vi "Actor Core.vi"(8 "error in":errorcluster, 11 "Nested in":refnum<class "UI.lvclass">) -> (0 "error out":errorcluster, 3 "Actor out":refnum<class "Actor.lvclass">)   [LabVIEW 2020, in "UI.lvlib" / "UI.lvclass"]
doc: "(<B>Filename</B>: Actor Framework.lvlib:Actor.lvclass:Actor Core.vi)\n\nReceives messages to the actor, reacts to them, and initiates any error handling that may shut the actor down.\n\nDescendant classes may override this VI to append parallel tasks for the actor to complete while it handles messages. Overrides use the Call Parent Method node."
uses:
  UI.lvclass
  <vilib>/ActorFramework/Actor/Actor.lvclass
  <vilib>/ActorFramework/Stop Msg/Stop Msg.lvclass
  Monedas/Monedas.lvclass
  Productos/Productos.lvclass
  Mensajes/Mensajes.lvclass
panel:
  out "String":string
  out "Dinero 2":dbl
  out "Dinero":dbl
  out "Costo":dbl
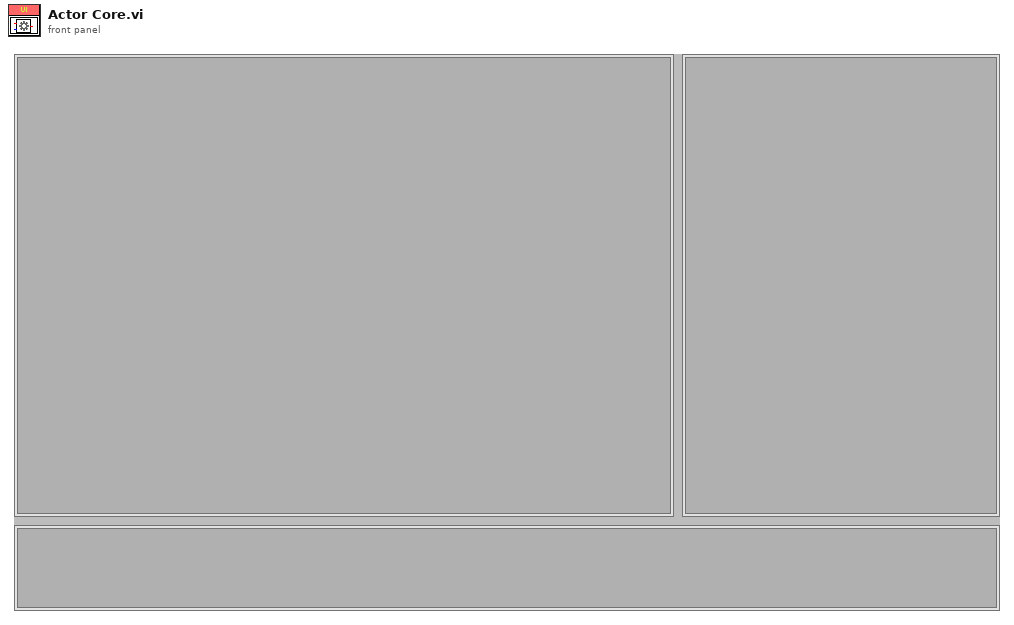
[diagram p1: front panel]
types:
  T1 = cluster{"Stop":refnum<user-event>, "Costo":refnum<user-event>, "Costo 2":refnum<user-event>, "Dinero":refnum<user-event>, "Dinero 2":refnum<user-event>, "String":refnum<user-event>, "String 2":refnum<user-event>}
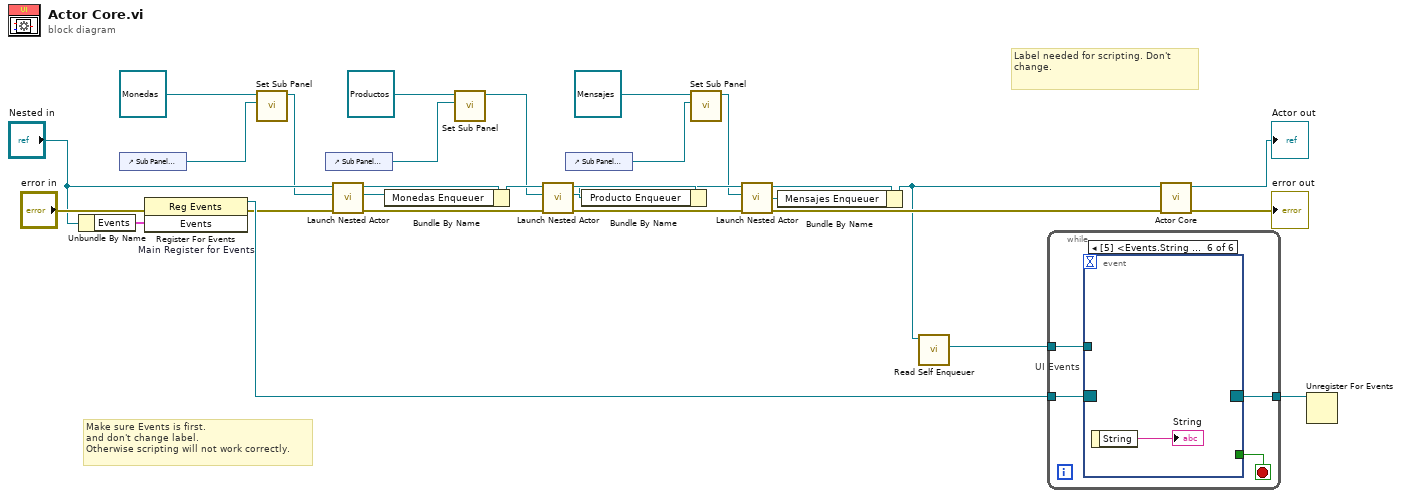
[diagram p0: block diagram]
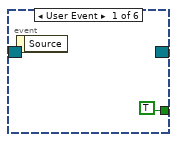
[diagram p2: hidden frame]
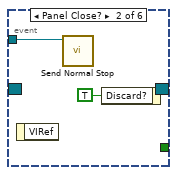
[diagram p3: hidden frame]
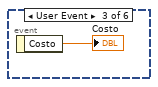
[diagram p4: hidden frame]
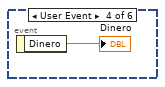
[diagram p5: hidden frame]
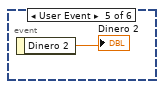
[diagram p6: hidden frame]
diagram:
  # "Label needed for scripting. Don't change."
  # "Make sure Events is first.\nand don't change label.\nOtherwise scripting will not work correctly."
  n1 = Unbundle By Name("Nested in") -> ("Events"=w27:T1)
  n2 = control-ref of="Sub Panel Monedas"() -> (w20:refnum<vi>)
  n3 = register-events "Main Register for Events"(error in="error in", w27) -> (reference out=w28:refnum<event-registration>, error out=w23:errorcluster)  [unwired: 1 in]
  n4 = call "Set Sub Panel.vi"("Sub Panel"=w20, "Monedas in"=refnum<class "Monedas.lvclass"> refnum ("Monedas.lvlib:Monedas.lvclass")) -> ("Monedas out"=w19:refnum<class "Monedas.lvclass">)  [unwired: 8 in, 1 out]
  n5 = control-ref of="Sub Panel Proucto"() -> (w17:refnum<vi>)
  n6 = call <vilib>:"Launch Nested Actor.vi"("error in (no error)"=w23, "Nested Actor"=w19, "Caller Actor in"="Nested in") -> ("error out"=w14:errorcluster, "Nested Actor's Enqueuer"=w10:refnum<class "Message Enqueuer.lvclass">, "Caller Actor out"=w11:refnum<class "UI.lvclass">)  [unwired: 6 in]
  n7 = Bundle By Name(cluster=w11, "Monedas Enqueuer"=w10) -> (w16:refnum<class "UI.lvclass">)
  n8 = call "Set Sub Panel.vi"("Sub Panel"=w17, "Productos in"=refnum<class "Productos.lvclass"> refnum ("Productos.lvlib:Productos.lvclass")) -> ("Productos out"=w13:refnum<class "Productos.lvclass">)  [unwired: 8 in, 1 out]
  n9 = call <vilib>:"Launch Nested Actor.vi"("error in (no error)"=w14, "Nested Actor"=w13, "Caller Actor in"=w16) -> ("error out"=w7:errorcluster, "Nested Actor's Enqueuer"=w12:refnum<class "Message Enqueuer.lvclass">, "Caller Actor out"=w15:refnum<class "UI.lvclass">)  [unwired: 6 in]
  n10 = control-ref of="Sub Panel Mensajes"() -> (w4:refnum<vi>)
  n11 = Bundle By Name(cluster=w15, "Producto Enqueuer"=w12) -> (w9:refnum<class "UI.lvclass">)
  n12 = call "Set Sub Panel.vi"("Sub Panel"=w4, "Mensajes in"=refnum<class "Mensajes.lvclass"> refnum ("Mensajes.lvlib:Mensajes.lvclass")) -> ("Mensajes out"=w3:refnum<class "Mensajes.lvclass">)  [unwired: 8 in, 1 out]
  n13 = call <vilib>:"Launch Nested Actor.vi"("error in (no error)"=w7, "Nested Actor"=w3, "Caller Actor in"=w9) -> ("error out"=w6:errorcluster, "Nested Actor's Enqueuer"=w1:refnum<class "Message Enqueuer.lvclass">, "Caller Actor out"=w8:refnum<class "UI.lvclass">)  [unwired: 6 in]
  n14 = Bundle By Name(cluster=w8, "Mensajes Enqueuer"=w1) -> (w2:refnum<class "UI.lvclass">)
  n15 = call <vilib>:"Read Self Enqueuer.vi"("Actor"=w2) -> ("Self Enqueuer"=w25:refnum<class "Message Enqueuer.lvclass">)  [unwired: 10 in]
  n16 = while {
    tunnel: w28 -> [w34]
    tunnel: [w32] -> w26
    tunnel: w25 -> [w31]
    stop <- w33 stop-if-true
    n17 = event "UI Events" shown="[5] <Events.String 2>: User Event" {
      selector: w34 -> [_ _ _ _ _ _]
      dyn-events: [_ _ _ _ _ _] -> w32
      timeout: _ -> [_ _ _ _ _ _]
      tunnel: [TRUE _ _ _ _ _] -> w33
      tunnel: w31 -> [_ w36 _ _ _ _]
      event User Event {
        n18 = event-data() -> ()  [unwired: 1 in, 1 out]
      }
      event Panel Close? {
        n19 = event-data() -> ()  [unwired: 1 in, 1 out]
        n20 = call <vilib>:"Send Normal Stop.vi"("Message Enqueuer"=w36) -> ()  [unwired: 10 in, 1 out]
        n21 = event-data("Discard?"=TRUE) -> ()  [unwired: 1 in, 1 out]
      }
      event User Event {
        n22 = event-data() -> ("Costo"=→"Costo":dbl)  [unwired: 1 in]
      }
      event User Event {
        n23 = event-data() -> ("Dinero"=→"Dinero":dbl)  [unwired: 1 in]
      }
      event User Event {
        n24 = event-data() -> ("Dinero 2"=→"Dinero 2":dbl)  [unwired: 1 in]
      }
      event User Event {
        n25 = event-data() -> ("String"=→"String":string)  [unwired: 1 in]
      }
    }
  }
  n26 = call-parent "Actor Core.vi"("error in"=w6, "Actor in"=w2) -> ("error out"=→"error out":errorcluster, "Actor out"=→"Actor out":refnum<class "Actor.lvclass">)  [unwired: 8 in]
  n27 = Unregister For Events(event registration refnum=w26) -> ()  [unwired: 1 in, 1 out]
